vi "SP_DS.vi"(3 "Commands":string[](array[string])) -> (1 "Commands Out":string[](array[string]))   [LabVIEW 2009]
panel:
  # "This LabVIEW item is deprecated.\n\nIt is believed to be unused and will be removed in a future version of SRV."
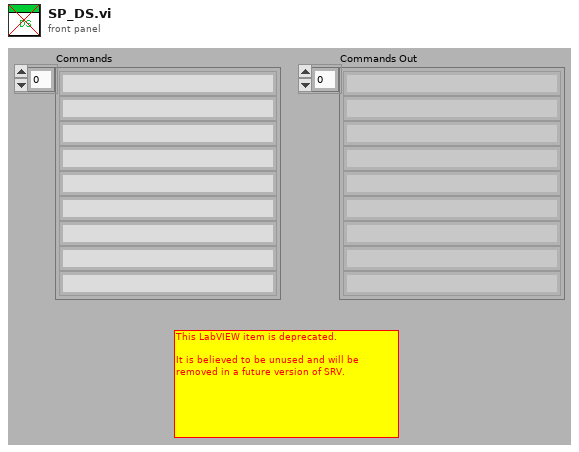
[diagram p1: front panel]
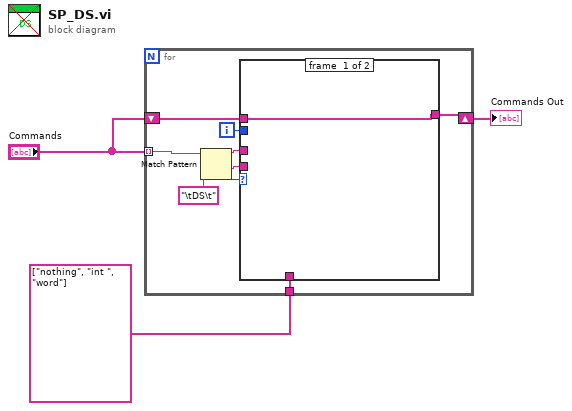
[diagram p0: block diagram]
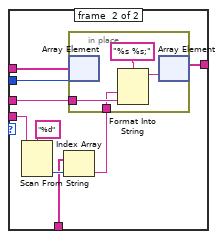
[diagram p2: hidden frame]
diagram:
  n1 = for {
    tunnel: "Commands" -> [w7] mode=indexing
    tunnel: string[] ["nothing", "int ", "word"] -> [w8]
    shift-right: [w4] -> w1
    shift-left: "Commands" -> [w6]
    i -> [w5]
    n2 = Match Pattern(string=w7, regular expression="\tDS\t") -> (before substring=w10:string, after substring=w9:string, offset past match=w11:i32)  [unwired: 1 in, 1 out]
    n3 = case shown="Default" w11 {
      tunnel: w10 -> [_ w17]
      tunnel: w9 -> [_ w20]
      tunnel: w8 -> [_ w21]
      tunnel: w6 -> [w13 w18]
      tunnel: w5 -> [_ w15]
      tunnel: [w13 w14] -> w4
      frame #0 {
      }
      frame #1 {
        n4 = Scan From String(format string="%d" ("regular expression"), input string=w20) -> (output 1=w22:i32)  [unwired: 3 in, 3 out]
        n5 = Index Array(array=w21, index=w22) -> (element=w16:string)
        n6 = in-place {
          in-place-border: w17 -> [w25]
          in-place-border: w16 -> [w24]
          n7 = in-place-array #1(w18, w15) -> ()  [unwired: 1 out]
          n8 = Format Into String(format string="%s %s;", w24, w25) -> (resulting string=w23:string)  [unwired: 2 in, 1 out]
          n9 = in-place-array #1(w23) -> (w14:string[])  [unwired: 1 out]
        }
      }
    }
  }
  "Commands Out" <- w1
